vi "HDF5_Write_AI_Record.vi"(8 "error in":errorcluster, 10 "AI_Data":T3, 11 "AI_Refs":T1 {"BlowerPwr_dset" format="%.0x"; "ElStdDev_dset" format="%.0x"; "AzStdDev_dset" format="%.0x"; "AI19_dset" format="%.0x"; "AI18_dset" format="%.0x"; "AI17_dset" format="%.0x"; "AI16_dset" format="%.0x"; "AI6_dset" format="%.0x"; "AI5_dset" format="%.0x"; "AI4_dset" format="%.0x"; "AI3_dset" format="%.0x"; "AI2_dset" format="%.0x"; "AI0_dset" format="%.0x"; "AI1_dset" format="%.0x"; "TimeString_dset" format="%.0x"; "TimeStamp_dset" format="%.0x"; "Group_ref" format="%.0x"}) -> (0 "error out":errorcluster, 2 "date/time string":string, 3 "current time":timestamp)   [LabVIEW 2018]
doc: "Write a single AI record with timestamp:\nAI\n AI_Info - cluster with Timestamp and other metadata for this record\n AI - 32 element Double array, up to 32 channels of AI data."
uses:
  Controls/Clusts/AI_Clust.ctl
  HDF5_AI_refs.ctl
  <vilib>/addons/h5labview2/base/hid_t.ctl
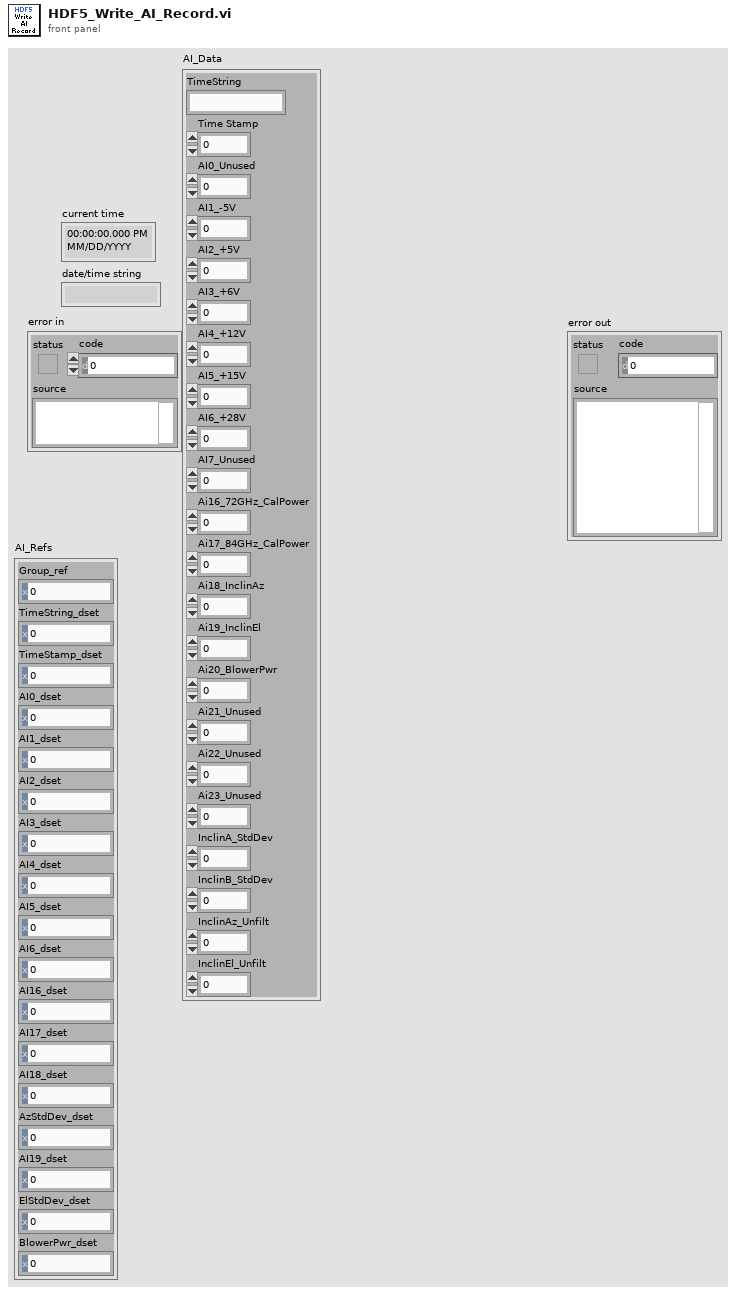
[diagram p1: front panel]
types:
  T1 = typedef "HDF5_AI_refs.ctl" = cluster{"Group_ref":T2, "TimeString_dset":T2, "TimeStamp_dset":T2, "AI0_dset":T2, "AI1_dset":T2, "AI2_dset":T2, "AI3_dset":T2, "AI4_dset":T2, "AI5_dset":T2, "AI6_dset":T2, "AI16_dset":T2, "AI17_dset":T2, "AI18_dset":T2, "AzStdDev_dset":T2, "AI19_dset":T2, "ElStdDev_dset":T2, "BlowerPwr_dset":T2}
  T2 = typedef "hid_t.ctl" = i32
  T3 = typedef "AI_Clust.ctl" = cluster{"TimeString":string, "Time Stamp":dbl, "AI0_Unused":dbl, "AI1_-5V":dbl, "AI2_+5V":dbl, "AI3_+6V":dbl, "AI4_+12V":dbl, "AI5_+15V":dbl, "AI6_+28V":dbl, "AI7_Unused":dbl, "Ai16_72GHz_CalPower":dbl, "Ai17_84GHz_CalPower":dbl, "Ai18_InclinAz":dbl, "Ai19_InclinEl":dbl, "Ai20_BlowerPwr":dbl, "Ai21_Unused":dbl, "Ai22_Unused":dbl, "Ai23_Unused":dbl, "InclinA_StdDev":dbl, "InclinB_StdDev":dbl, "InclinAz_Unfilt":dbl, "InclinEl_Unfilt":dbl}
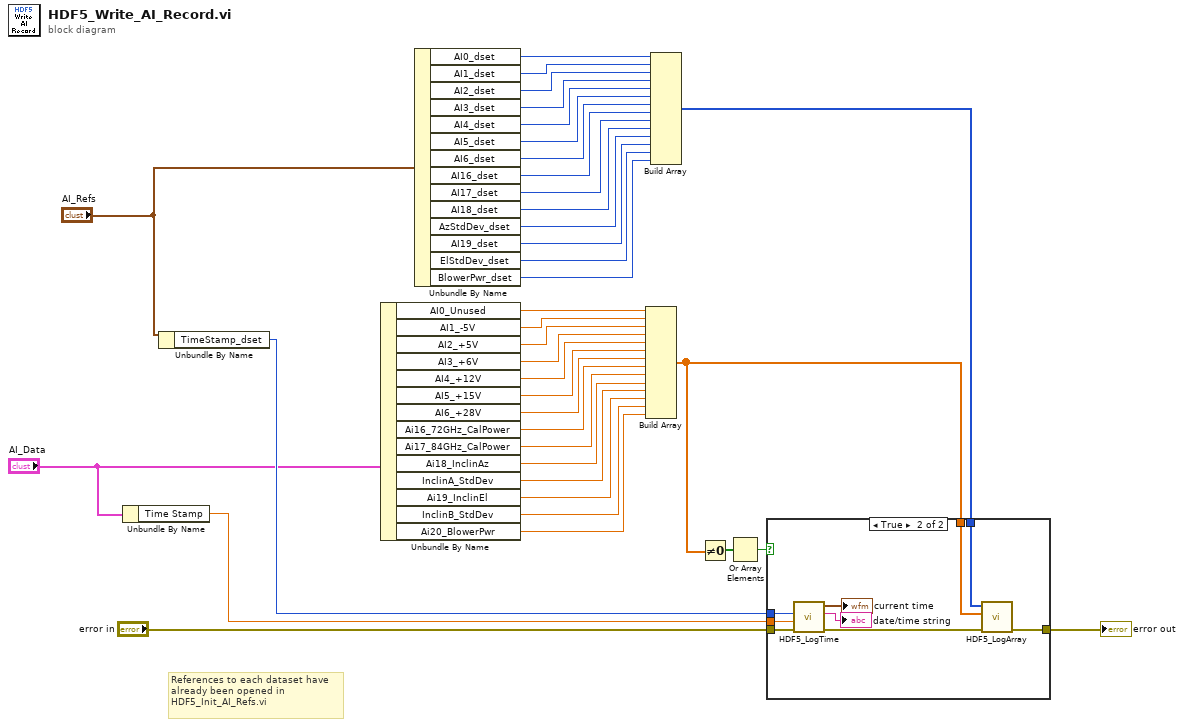
[diagram p0: block diagram]
diagram:
  # "References to each dataset have \nalready been opened in \nHDF5_Init_AI_Refs.vi"
  n1 = Unbundle By Name("AI_Data") -> ("Time Stamp"=w4:dbl)
  n2 = Unbundle By Name("AI_Refs") -> ("TimeStamp_dset"=w38:T2)
  n3 = Unbundle By Name("AI_Data") -> ("AI0_Unused"=w19:dbl, "AI1_-5V"=w20:dbl, "AI2_+5V"=w21:dbl, "AI3_+6V"=w22:dbl, "AI4_+12V"=w23:dbl, "AI5_+15V"=w24:dbl, "AI6_+28V"=w25:dbl, "Ai16_72GHz_CalPower"=w26:dbl, "Ai17_84GHz_CalPower"=w27:dbl, "Ai18_InclinAz"=w15:dbl, "InclinA_StdDev"=w11:dbl, "Ai19_InclinEl"=w14:dbl, "InclinB_StdDev"=w10:dbl, "Ai20_BlowerPwr"=w7:dbl)
  n4 = Unbundle By Name("AI_Refs") -> ("AI0_dset"=w37:T2, "AI1_dset"=w36:T2, "AI2_dset"=w35:T2, "AI3_dset"=w34:T2, "AI4_dset"=w33:T2, "AI5_dset"=w32:T2, "AI6_dset"=w31:T2, "AI16_dset"=w30:T2, "AI17_dset"=w29:T2, "AI18_dset"=w13:T2, "AzStdDev_dset"=w9:T2, "AI19_dset"=w12:T2, "ElStdDev_dset"=w8:T2, "BlowerPwr_dset"=w6:T2)
  n5 = Build Array(w19, w20, w21, w22, w23, w24, w25, w26, w27, w15, w11, w14, w10, w7) -> (w1:dbl[])
  n6 = Build Array(w37, w36, w35, w34, w33, w32, w31, w30, w29, w13, w9, w12, w8, w6) -> (w28:T2[])
  n7 = Not Equal To 0?(x=w1) -> (x != 0?=w3:bool[])
  n8 = Or Array Elements(Boolean array=w3) -> (logical OR=w2:bool)
  n9 = case shown="True" w2 {
    tunnel: w38 -> [_ w48]
    tunnel: w28 -> [_ w46]
    tunnel: w1 -> [_ w45]
    tunnel: [w39 w42] -> w18
    tunnel: "error in" -> [w39 w41]
    tunnel: w4 -> [_ w40]
    frame False {
      # "Don't log if all values are zero."
    }
    frame True {
      n10 = call "HDF5_LogTime.vi"("error in (no error)"=w41, "Timestamp"=w40, "TimeStamp_dset"=w48) -> ("error out"=w47:errorcluster, "date/time string"=→"date/time string":string, "current time"=→"current time":timestamp)  [unwired: 6 in]
      n11 = call "HDF5_LogArray.vi"("error in (no error)"=w47, "array of Data"=w45, "array of Refs"=w46) -> ("error out"=w42:errorcluster)  [unwired: 8 in]
    }
  }
  "error out" <- w18
